vi "AccessLog写入.vi"(11 "Log":string) -> ()   [LabVIEW 2016, in "斯坦道总氮.lvlib"]
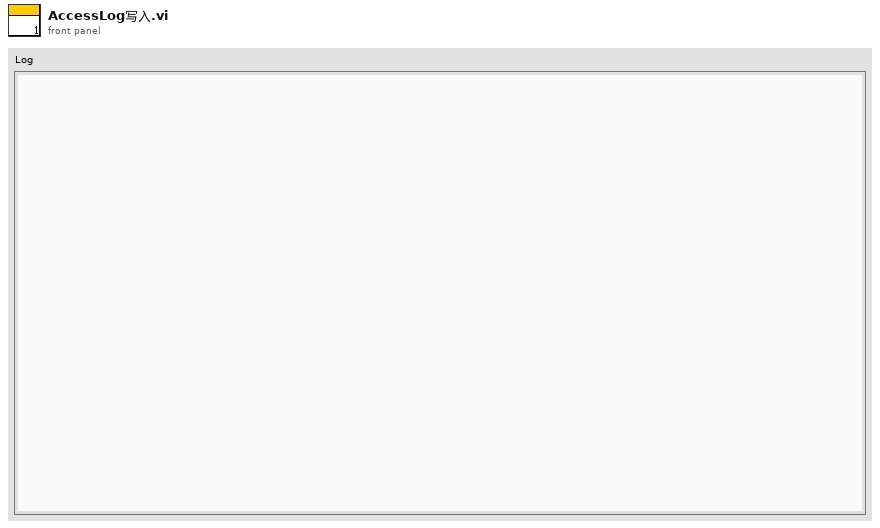
[diagram p1: front panel]
types:
  T1 = enum16{"open", "replace", "create", "open or create", "replace or create", "replace or create with confirmation"}
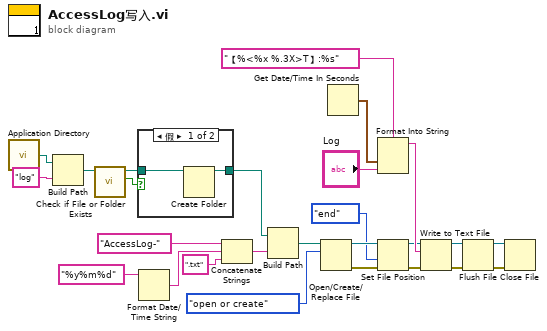
[diagram p0: block diagram]
diagram:
  n1 = call <vilib>:"Application Directory.vi"() -> ("Application Directory"=w4:path)
  n2 = Build Path(base path=w4, name or relative path="log" ("名称或相对路径")) -> (appended path=w2:path)
  n3 = call <vilib>:"Check if File or Folder Exists.vi"("path"=w2) -> ("file or folder exists?"=w17:bool, "dup path"=w16:path)  [unwired: 8 in, 1 out]
  n4 = case shown="假" w17 {
    tunnel: w16 -> [w28 w29]
    tunnel: [w27 w29] -> w15
    frame False {
      n5 = Create Folder(path (use dialog)=w28) -> (created path=w27:path)  [unwired: 2 in, 2 out]
    }
    frame True {
    }
  }
  n6 = Format Date/Time String(time format string (%c)="%y%m%d" ("时间格式字符串(%c)")) -> (date/time string=w13:string)  [unwired: 2 in]
  n7 = Concatenate Strings("AccessLog-" ("字符串"), w13, ".txt" ("字符串")) -> (w12:string)
  n8 = Build Path(base path=w15, name or relative path=w12) -> (appended path=w11:path)
  n9 = Open/Create/Replace File(file path (use dialog)=w11, operation (0:open)=T1."open or create" ("操作(0:open)")) -> (refnum out=w19:refnum<file>, error out=w21:errorcluster)  [unwired: 4 in, 1 out]
  n10 = Get Date/Time In Seconds() -> (seconds since 1Jan1904=w25:timestamp)
  n11 = Format Into String(format string="【%<%x %.3X>T】:%s" ("格式字符串"), w25, "Log") -> (resulting string=w24:string)  [unwired: 2 in, 1 out]
  n12 = Set File Position(refnum=w19, from (0:start)=enum16{"start", "end", "current"}."end" ("自（0:起始）"), error in=w21) -> (refnum out=w20:refnum<file>, error out=w22:errorcluster)  [unwired: 1 in]
  n13 = Write to Text File(file (use dialog)=w20, text=w24, error in=w22) -> (refnum out=w7:refnum<file>, error out=w6:errorcluster)  [unwired: 1 in, 1 out]
  n14 = Flush File(refnum=w7, error in=w6) -> (refnum out=w9:refnum<file>, error out=w8:errorcluster)
  n15 = Close File(refnum=w9, error in=w8) -> ()  [unwired: 2 out]
